vi "Handle Error.vi"(8 "error in (no error)":errorcluster, 11 "Chat Window in":refnum<class "Chat Window.lvclass">) -> (0 "error out":errorcluster, 2 "stop actor?":bool=TRUE, 3 "Chat Window out":refnum<class "Chat Window.lvclass">)   [LabVIEW 2020, in "Chat Window.lvlib" / "Chat Window.lvclass"]
doc: "(<B>Filename</B>: Actor Framework.lvlib:Actor.lvclass:Handle Error.vi)\n\nDefines how the actor handles an error that occurred while processing a message. By default, this method does nothing except stop the actor."
uses:
  Chat Window.lvclass
  <vilib>/ActorFramework/Actor/Actor.lvclass
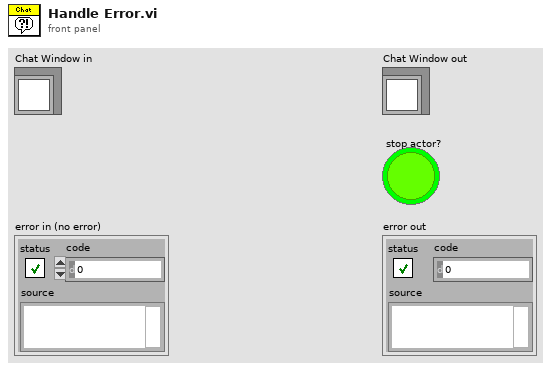
[diagram p1: front panel]
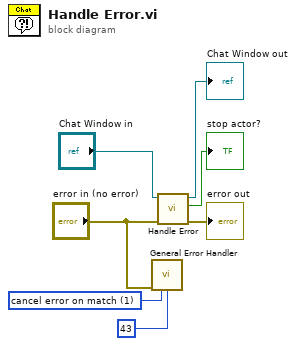
[diagram p0: block diagram]
diagram:
  w1 = 1 items=["no exception", "cancel error on match", "set error on match"] ("[exception action] (none:0)")
  n1 = call <vilib>:"General Error Handler.vi"("error in (no error)"="error in (no error)", "[exception action] (none:0)"=w1, "[exception code]"=43) -> ()  [unwired: 8 in, 5 out]
  n2 = call-parent "Handle Error.vi"("error in (no error)"="error in (no error)", "Actor in"="Chat Window in") -> ("error out"=→"error out":errorcluster, "stop actor?"=→"stop actor?":bool, "Actor out"=→"Chat Window out":refnum<class "Chat Window.lvclass">)  [unwired: 7 in]
